vi "Force Update.vi"(7 "Update Origin":bool, 9 "All Controls and Decorations":bool, 10 "Value and Position":refnum<vi>[](array[refnum]), 11 "VI Refnum":refnum<vi>) -> ()   [LabVIEW 2015, in "Front Panel Publisher.lvlib"]
doc: "This VI will force controls passed in to the <b>Value and Position</b> to have their current value, along with any attributes sent to all active connections to the web page. Optionally the <b>All Controls and Decorations</b> can be used which will just update the whole panel with new attributes and values."
uses:
  Front Panel Publisher.lvlib
  Front Panel Manager_class/Front Panel Manager.lvclass
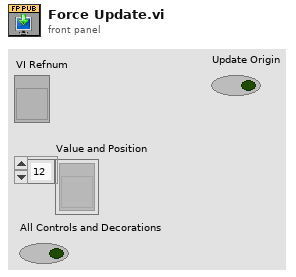
[diagram p1: front panel]
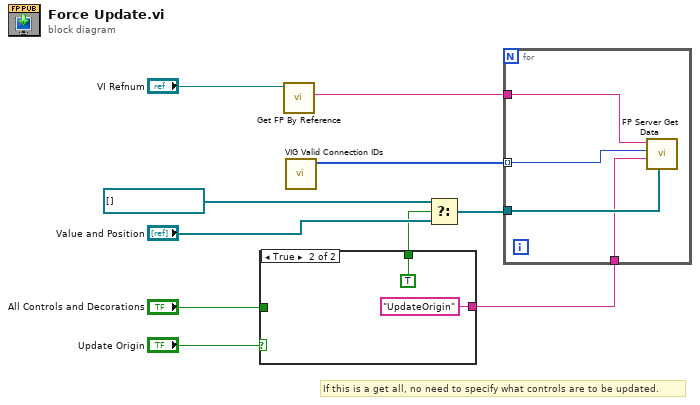
[diagram p0: block diagram]
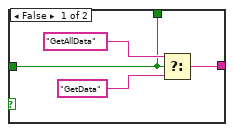
[diagram p2: hidden frame]
diagram:
  # "If this is a get all, no need to specify what controls are to be updated."
  n1 = case shown="True" "Update Origin" {
    tunnel: [w12 "UpdateOrigin" ("Message")] -> w7
    tunnel: "All Controls and Decorations" -> [w11 _]
    tunnel: [w11 TRUE ("All Controls and Decorations")] -> w1
    frame False {
      n2 = Select(t="GetAllData" ("Message"), s=w11, f="GetData" ("Message")) -> (s? t:f=w12:string)
    }
    frame True {
    }
  }
  n3 = call "Get FP By Reference.vi"("VI Refnum"="VI Refnum") -> ("WFP Name"=w8:string)  [unwired: 7 in, 3 out]
  n4 = call "VIG Valid Connection IDs.vi"() -> ("Connections"=w9:u64[])  [unwired: 8 in, 3 out]
  n5 = Select(t=refnum<vi>[] [], s=w1, f="Value and Position") -> (s? t:f=w5:refnum<vi>[])
  n6 = for {
    tunnel: w9 -> [w19] mode=indexing
    tunnel: w8 -> [w20]
    tunnel: w5 -> [w18]
    tunnel: w7 -> [w17]
    n7 = call "FP Server Get Data.vi"("Values and Position"=w18, "Message"=w17, "Connection ID"=w19, "Page"=w20) -> ()  [unwired: 7 in, 1 out]
  }
